vi "Load Target.vi"(6 "Number of Bits (n)":u32, 8 "error in":errorcluster, 9 "Target":dbl, 10 "IChromosome Type":refnum<class "IChromosome.lvclass">, 11 "IPopulation in":refnum<class "IPopulation.lvclass">) -> (0 "error out":errorcluster, 3 "IPopulation out":refnum<class "IPopulation.lvclass">)   [LabVIEW 2016, in "IPopulation.lvclass"]
uses:
  IPopulation.lvclass
  IChromosome/IChromosome.lvclass
  IPopulation.lvclass/IPopulation.ctl
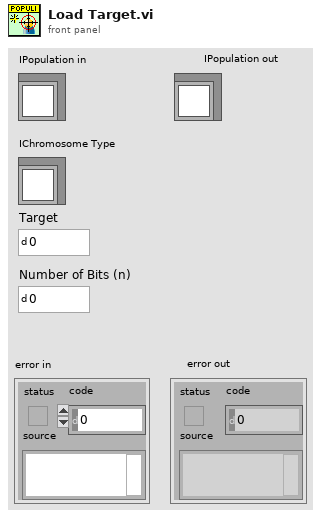
[diagram p1: front panel]
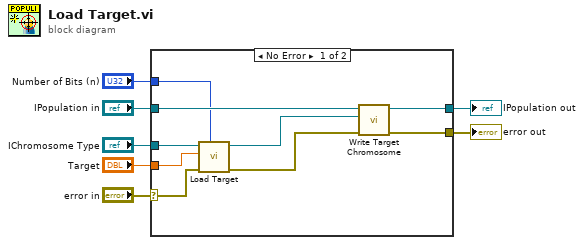
[diagram p0: block diagram]
diagram:
  n1 = case shown="No Error" "error in" {
    selector: "error in" -> [w10 w18]
    tunnel: [w8 w18] -> w6
    tunnel: [w15 w17] -> w4
    tunnel: "IPopulation in" -> [w16 w17]
    tunnel: "Target" -> [w13 _]
    tunnel: "IChromosome Type" -> [w12 _]
    tunnel: "Number of Bits (n)" -> [w11 _]
    frame No Error {
      n2 = call "Load Target.vi"("Number of Bits (n)"=w11, "error in"=w10, "Target"=w13, "IChromosome Type"=w12) -> ("error out"=w9:errorcluster, "Target Chromosome Out"=w14:refnum<class "IChromosome.lvclass">)  [unwired: 6 in]
      n3 = call "Write Target Chromosome.vi"("error in (no error)"=w9, "IChromosome.lvclass"=w14, "IPopulation in"=w16) -> ("error out"=w8:errorcluster, "IPopulation out"=w15:refnum<class "IPopulation.lvclass">)  [unwired: 7 in]
    }
    frame Error {
    }
  }
  "error out" <- w6
  "IPopulation out" <- w4
